vi "Compare to Accel Distances.vi"(5 "dA":dbl, 6 "Sample Period (s)":dbl, 7 "Values":cluster{"accel":dbl, "velocity":dbl}, 8 "Speeds in":T1={"maxV (fps)"=20.0, "Accel Limit (fps^2)"=20.0, "Initial V (fps)"=0.0, "Sample Period (s)"=0.02, "Jerk Limit (fps^3)"=0.0, "Distances"=[]}, 10 "Current  Length":dbl, 11 "Total Segment Length":dbl) -> (0 "End Loop":bool, 1 "Ends":cluster{"Accel End":bool, "Decel End":bool}, 2 "Values out":cluster{"accel":dbl, "velocity":dbl}, 3 "Action":enum16{"Const", "Accel", "Decel", "Both"}(ring))   [LabVIEW 2025]
uses:
  Types/Speeds.ctl
panel:
  out "Accel Action":enum16{"Const", "Accel", "Decel", "Both"}(ring)
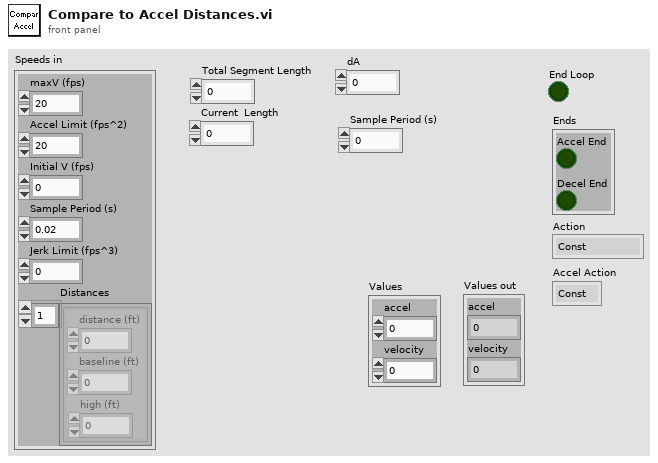
[diagram p1: front panel]
types:
  T1 = typedef "Speeds.ctl" = cluster{"maxV (fps)":dbl, "Accel Limit (fps^2)":dbl, "Initial V (fps)":dbl, "Sample Period (s)":dbl, "Jerk Limit (fps^3)":dbl, "Distances":cluster{"distance (ft)":dbl, "baseline (ft)":dbl, "high (ft)":dbl}[]}
  T2 = cluster{"distance (ft)":dbl, "baseline (ft)":dbl, "high (ft)":dbl}[]
  T3 = cluster{"distance (ft)":dbl, "baseline (ft)":dbl, "high (ft)":dbl}
  T4 = cluster{"distance (ft)":bool, "baseline (ft)":bool, "high (ft)":bool}
  T5 = cluster{"Accel Limit (fps^2)":dbl, "maxV (fps)":dbl}
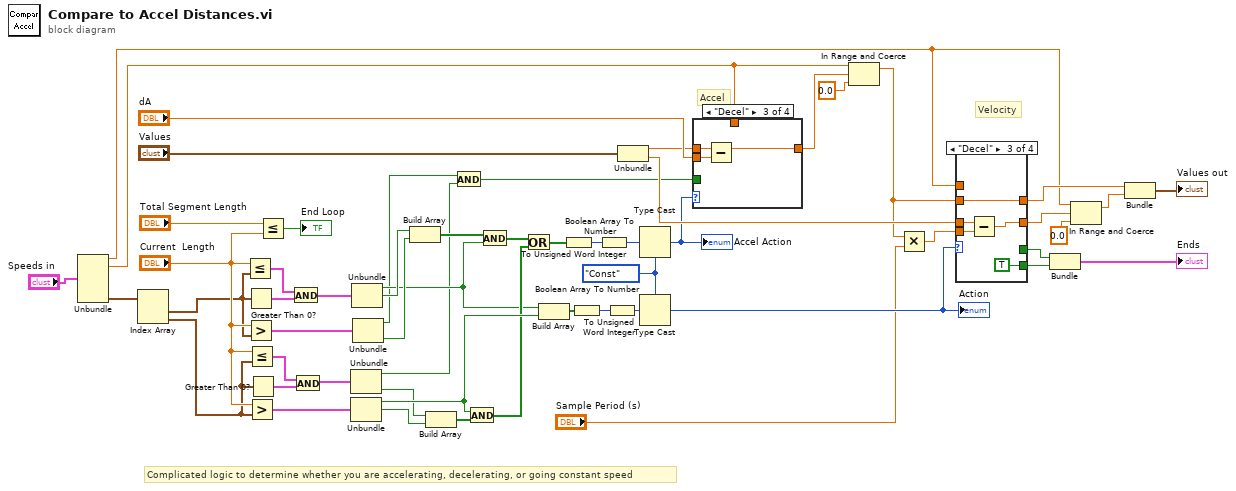
[diagram p0: block diagram]
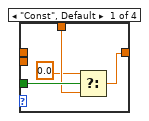
[diagram p2: hidden frame]
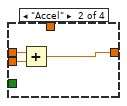
[diagram p3: hidden frame]
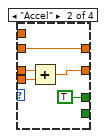
[diagram p6: hidden frame]
diagram:
  w35 = enum16{"Const", "Accel", "Decel", "Both"}."Const" ("Action")
  # "Complicated logic to determine whether you are accelerating, decelerating, or going constant speed"
  # "Accel"
  # "Velocity"
  n1 = Unbundle("Speeds in") -> ("maxV (fps)"=w2:dbl, "Accel Limit (fps^2)"=w12:dbl, "Distances"=w3:T2)  [unwired: 3 out]
  n2 = Index Array(array=w3) -> (element #1=w5:T3, element #2=w4:T3)  [unwired: 2 in]
  n3 = Less Or Equal?(x="Current  Length", y=w5) -> (x <= y?=w53:T4)
  n4 = Greater Than 0?(x=w5) -> (x > 0?=w54:T4)
  n5 = Greater?(x="Current  Length", y=w5) -> (0:w34:T4)
  n6 = Less Or Equal?(x="Current  Length", y=w4) -> (x <= y?=w33:T4)
  n7 = Greater?(x="Current  Length", y=w4) -> (0:w41:T4)
  n8 = Greater Than 0?(x=w4) -> (x > 0?=w32:T4)
  n9 = Less Or Equal?(x="Total Segment Length", y="Current  Length") -> (x <= y?=→"End Loop":bool)
  n10 = And(x=w53, y=w54) -> (x .and. y?=w42:T4)
  n11 = And(x=w33, y=w32) -> (x .and. y?=w29:T4)
  n12 = Unbundle(w29) -> ("distance (ft)"=w7:bool, "high (ft)"=w19:bool)  [unwired: 1 out]
  n13 = Unbundle(w41) -> ("distance (ft)"=w28:bool, "baseline (ft)"=w20:bool)  [unwired: 1 out]
  n14 = Unbundle(w42) -> ("distance (ft)"=w23:bool, "baseline (ft)"=w26:bool)  [unwired: 1 out]
  n15 = Unbundle(w34) -> ("distance (ft)"=w9:bool, "high (ft)"=w30:bool)  [unwired: 1 out]
  n16 = Build Array(w26, w30) -> (w22:bool[])
  n17 = Build Array(w19, w20) -> (w27:bool[])
  n18 = And(x=w9, y=w7) -> (x .and. y?=w8:bool)
  n19 = And(x=w28, y=w27) -> (x .and. y?=w25:bool[])
  n20 = And(x=w22, y=w23) -> (x .and. y?=w21:bool[])
  n21 = Or(x=w21, y=w25) -> (x .or. y?=w24:bool[])
  n22 = Build Array(w23, w28) -> (w43:bool[])
  n23 = Boolean Array To Number(Boolean array=w24) -> (number=w38:u32)
  n24 = Boolean Array To Number(Boolean array=w43) -> (number=w52:u32)
  n25 = To Unsigned Word Integer(number=w38) -> (unsigned 16bit integer=w37:u16)
  n26 = To Unsigned Word Integer(number=w52) -> (unsigned 16bit integer=w40:u16)
  n27 = Unbundle("Values") -> ("accel"=w45:dbl, "velocity"=w44:dbl)
  n28 = Type Cast(type=w35, x=w37) -> (*(type *) &x=w36:enum16{"Const", "Accel", "Decel", "Both"})
  "Accel Action" <- w36
  n29 = Type Cast(type=w35, x=w40) -> (*(type *) &x=w39:enum16{"Const", "Accel", "Decel", "Both"})
  "Action" <- w39
  n30 = case shown="\"Decel\"" w36 {
    tunnel: w45 -> [_ w63 w66 w67]
    tunnel: [w57 w61 w64 w67] -> w14
    tunnel: "dA" -> [_ w62 w65 _]
    tunnel: w12 -> [w59 _ _ _]
    tunnel: w8 -> [w60 _ _ _]
    frame "Const", Default {
      n31 = Select(t=0.0, s=w60, f=w59) -> (s? t:f=w57:dbl)
    }
    frame "Accel" {
      n32 = Add(x=w63, y=w62) -> (x+y=w61:dbl)
    }
    frame "Decel" {
      n33 = Subtract(x=w66, y=w65) -> (x-y=w64:dbl)
    }
    frame "Both" {
    }
  }
  n34 = In Range and Coerce(upper limit=w12, x=w14, lower limit=0.0) -> (coerced(x)=w13:dbl)  [unwired: 1 out]
  n35 = Multiply(x=w13, y="Sample Period (s)") -> (x*y=w18:dbl)
  n36 = case shown="\"Decel\"" w39 {
    tunnel: w44 -> [w68 w74 w79 w81]
    tunnel: [w68 w72 w77 w81] -> w11
    tunnel: w18 -> [_ w73 w78 _]
    tunnel: [_ TRUE _ _] -> w49
    tunnel: [_ _ TRUE _] -> w48
    tunnel: [w69 w70 w75 w80] -> w10
    tunnel: w13 -> [w69 w70 w75 w80]
    tunnel: w2 -> [_ _ _ _]
    frame "Const", Default {
    }
    frame "Accel" {
      n37 = Add(x=w74, y=w73) -> (x+y=w72:dbl)
    }
    frame "Decel" {
      n38 = Subtract(x=w79, y=w78) -> (x-y=w77:dbl)
    }
    frame "Both" {
    }
  }
  n39 = Bundle(w49, w48) -> (→"Ends":cluster{bool, bool})  [unwired: 1 in]
  n40 = In Range and Coerce(upper limit=w2, x=w11, lower limit=0.0) -> (coerced(x)=w1:dbl)  [unwired: 1 out]
  n41 = Bundle("Accel Limit (fps^2)"=w10, "maxV (fps)"=w1) -> (→"Values out":T5)  [unwired: 1 in]
